vi "VI Tree.vi"   [LabVIEW 2009, in "Keithley 3700 Series.lvlib"]
doc: "This is the instrument driver for the <INSTRUMENT NAME>. The VI Tree displays all the user-callable VIs of the instrument driver in an organized table."
uses:
  <instrlib>/Keithley 3706/Keithley 3700 Series.lvlib
panel:
  # "(c) 2007 <Enter Company Name Here>.  ALL RIGHTS RESERVED."
  # "SEE DIAGRAM\nFOR VI TREE."
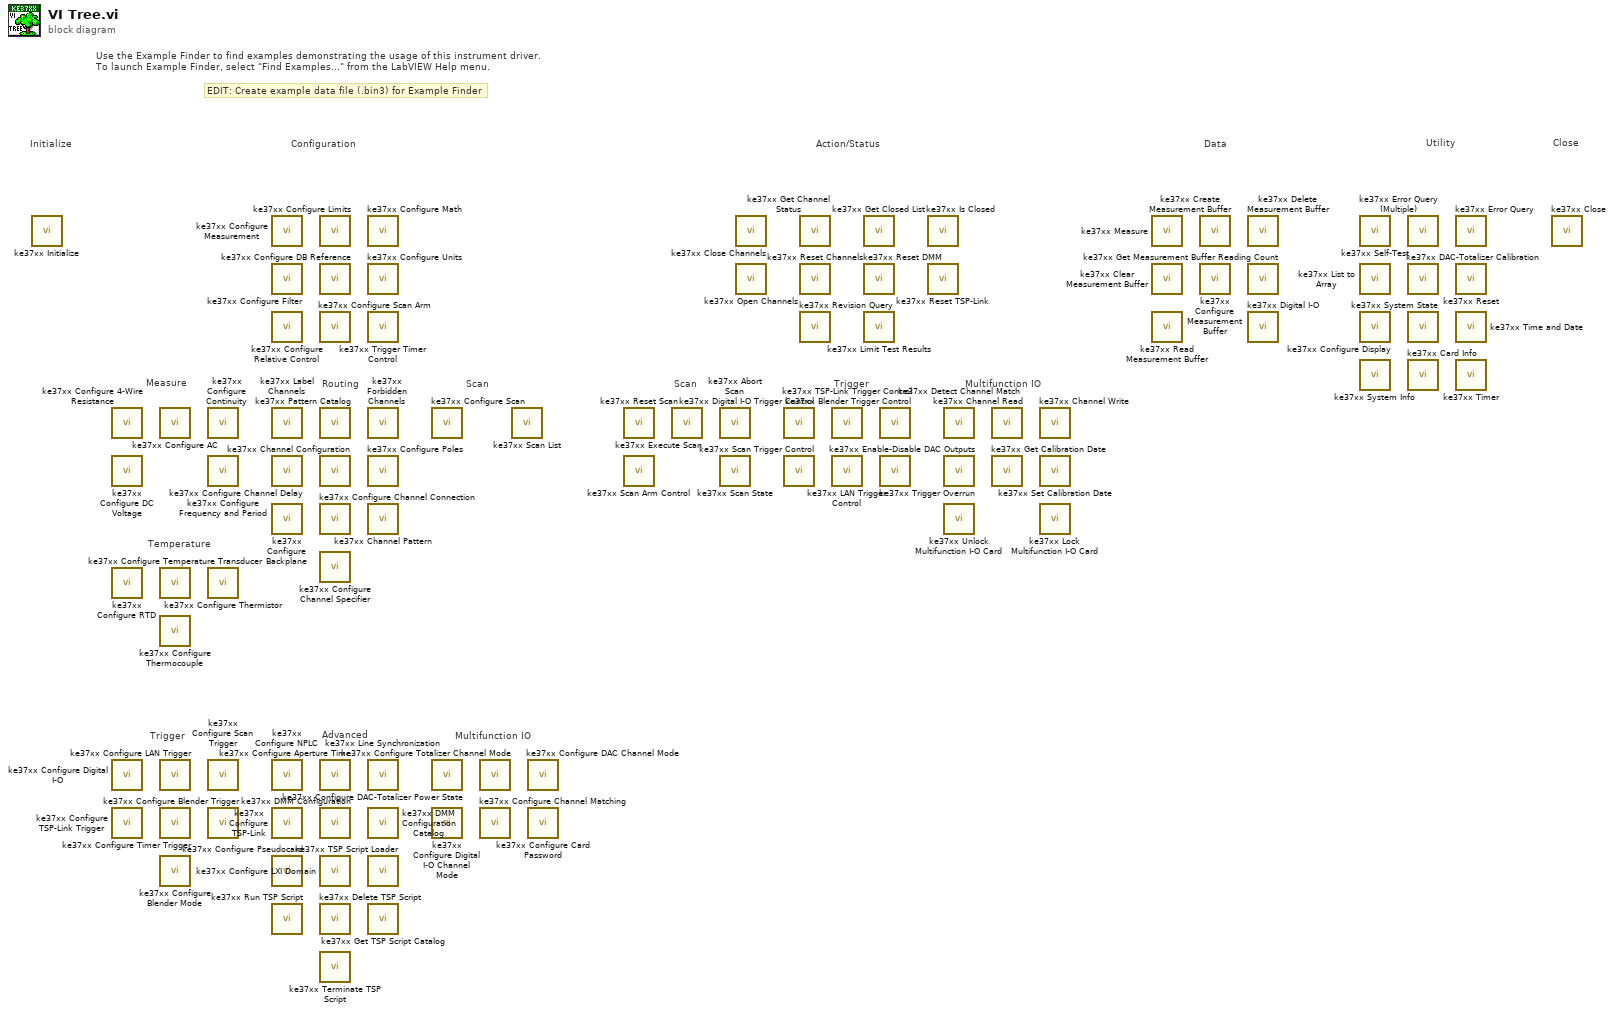
[diagram p0: block diagram]
diagram:
  # "Multifunction IO"
  # "Trigger"
  # "Scan"
  # "Multifunction IO"
  # "Advanced"
  # "Trigger"
  # "Scan"
  # "Routing"
  # "Temperature"
  # "Measure"
  # "EDIT: Create example data file (.bin3) for Example Finder"
  # "Use the Example Finder to find examples demonstrating the usage of this instrument driver.\nTo launch Example Finder, select \"Find Examples...\" from the LabVIEW Help menu."
  # "Configuration"
  # "Utility"
  # "Data"
  # "Action/Status"
  # "Close"
  # "Initialize"
  n1 = call <instrlib>:"ke37xx Initialize.vi"() -> ()  [unwired: 14 in, 2 out]
  n2 = call <instrlib>:"ke37xx Configure 4-Wire Resistance.vi"() -> ()  [unwired: 14 in, 2 out]
  n3 = call <instrlib>:"ke37xx Configure DC Voltage.vi"() -> ()  [unwired: 14 in, 2 out]
  n4 = call <instrlib>:"ke37xx Configure RTD.vi"() -> ()  [unwired: 14 in, 2 out]
  n5 = call <instrlib>:"ke37xx Configure Digital I-O.vi"() -> ()  [unwired: 14 in, 2 out]
  n6 = call <instrlib>:"ke37xx Configure TSP-Link Trigger.vi"() -> ()  [unwired: 14 in, 2 out]
  n7 = call <instrlib>:"ke37xx Configure AC.vi"() -> ()  [unwired: 14 in, 2 out]
  n8 = call <instrlib>:"ke37xx Configure Temperature Transducer.vi"() -> ()  [unwired: 14 in, 2 out]
  n9 = call <instrlib>:"ke37xx Configure Thermocouple.vi"() -> ()  [unwired: 14 in, 2 out]
  n10 = call <instrlib>:"ke37xx Configure LAN Trigger.vi"() -> ()  [unwired: 14 in, 2 out]
  n11 = call <instrlib>:"ke37xx Configure Timer Trigger.vi"() -> ()  [unwired: 14 in, 2 out]
  n12 = call <instrlib>:"ke37xx Configure Blender Mode.vi"() -> ()  [unwired: 14 in, 2 out]
  n13 = call <instrlib>:"ke37xx Configure Continuity.vi"() -> ()  [unwired: 14 in, 2 out]
  n14 = call <instrlib>:"ke37xx Configure Frequency and Period.vi"() -> ()  [unwired: 14 in, 2 out]
  n15 = call <instrlib>:"ke37xx Configure Thermistor.vi"() -> ()  [unwired: 14 in, 2 out]
  n16 = call <instrlib>:"ke37xx Configure Scan Trigger.vi"() -> ()  [unwired: 14 in, 2 out]
  n17 = call <instrlib>:"ke37xx Configure Blender Trigger.vi"() -> ()  [unwired: 14 in, 2 out]
  n18 = call <instrlib>:"ke37xx Configure Measurement.vi"() -> ()  [unwired: 14 in, 2 out]
  n19 = call <instrlib>:"ke37xx Configure Filter.vi"() -> ()  [unwired: 14 in, 2 out]
  n20 = call <instrlib>:"ke37xx Configure Relative Control.vi"() -> ()  [unwired: 14 in, 2 out]
  n21 = call <instrlib>:"ke37xx Label Channels.vi"() -> ()  [unwired: 14 in, 2 out]
  n22 = call <instrlib>:"ke37xx Configure Channel Delay.vi"() -> ()  [unwired: 14 in, 2 out]
  n23 = call <instrlib>:"ke37xx Configure Backplane.vi"() -> ()  [unwired: 14 in, 2 out]
  n24 = call <instrlib>:"ke37xx Configure NPLC.vi"() -> ()  [unwired: 14 in, 2 out]
  n25 = call <instrlib>:"ke37xx Configure TSP-Link.vi"() -> ()  [unwired: 14 in, 2 out]
  n26 = call <instrlib>:"ke37xx Configure Pseudocard.vi"() -> ()  [unwired: 14 in, 2 out]
  n27 = call <instrlib>:"ke37xx Run TSP Script.vi"() -> ()  [unwired: 10 in, 2 out]
  n28 = call <instrlib>:"ke37xx Configure Limits.vi"() -> ()  [unwired: 14 in, 2 out]
  n29 = call <instrlib>:"ke37xx Configure DB Reference.vi"() -> ()  [unwired: 14 in, 2 out]
  n30 = call <instrlib>:"ke37xx Configure Scan Arm.vi"() -> ()  [unwired: 14 in, 2 out]
  n31 = call <instrlib>:"ke37xx Pattern Catalog.vi"() -> ()  [unwired: 13 in, 3 out]
  n32 = call <instrlib>:"ke37xx Channel Configuration.vi"() -> ()  [unwired: 13 in, 3 out]
  n33 = call <instrlib>:"ke37xx Configure Channel Connection.vi"() -> ()  [unwired: 14 in, 2 out]
  n34 = call <instrlib>:"ke37xx Configure Channel Specifier.vi"() -> ()  [unwired: 13 in, 3 out]
  n35 = call <instrlib>:"ke37xx Configure Aperture Time.vi"() -> ()  [unwired: 14 in, 2 out]
  n36 = call <instrlib>:"ke37xx DMM Configuration.vi"() -> ()  [unwired: 13 in, 3 out]
  n37 = call <instrlib>:"ke37xx Configure LXI Domain.vi"() -> ()  [unwired: 14 in, 2 out]
  n38 = call <instrlib>:"ke37xx Delete TSP Script.vi"() -> ()  [unwired: 10 in, 2 out]
  n39 = call <instrlib>:"ke37xx Terminate TSP Script.vi"() -> ()  [unwired: 10 in, 2 out]
  n40 = call <instrlib>:"ke37xx Configure Math.vi"() -> ()  [unwired: 14 in, 2 out]
  n41 = call <instrlib>:"ke37xx Configure Units.vi"() -> ()  [unwired: 14 in, 2 out]
  n42 = call <instrlib>:"ke37xx Trigger Timer Control.vi"() -> ()  [unwired: 13 in, 3 out]
  n43 = call <instrlib>:"ke37xx Forbidden Channels.vi"() -> ()  [unwired: 13 in, 3 out]
  n44 = call <instrlib>:"ke37xx Configure Poles.vi"() -> ()  [unwired: 14 in, 2 out]
  n45 = call <instrlib>:"ke37xx Channel Pattern.vi"() -> ()  [unwired: 13 in, 3 out]
  n46 = call <instrlib>:"ke37xx Line Synchronization.vi"() -> ()  [unwired: 14 in, 2 out]
  n47 = call <instrlib>:"ke37xx DMM Configuration Catalog.vi"() -> ()  [unwired: 13 in, 3 out]
  n48 = call <instrlib>:"ke37xx TSP Script Loader.vi"() -> ()  [unwired: 14 in, 2 out]
  n49 = call <instrlib>:"ke37xx Get TSP Script Catalog.vi"() -> ()  [unwired: 9 in, 3 out]
  n50 = call <instrlib>:"ke37xx Configure Scan.vi"() -> ()  [unwired: 14 in, 2 out]
  n51 = call <instrlib>:"ke37xx Configure DAC-Totalizer Power State.vi"() -> ()  [unwired: 10 in, 2 out]
  n52 = call <instrlib>:"ke37xx Configure Digital I-O Channel Mode.vi"() -> ()  [unwired: 10 in, 2 out]
  n53 = call <instrlib>:"ke37xx Configure Totalizer Channel Mode.vi"() -> ()  [unwired: 10 in, 2 out]
  n54 = call <instrlib>:"ke37xx Configure Channel Matching.vi"() -> ()  [unwired: 14 in, 2 out]
  n55 = call <instrlib>:"ke37xx Scan List.vi"() -> ()  [unwired: 13 in, 3 out]
  n56 = call <instrlib>:"ke37xx Configure DAC Channel Mode.vi"() -> ()  [unwired: 10 in, 2 out]
  n57 = call <instrlib>:"ke37xx Configure Card Password.vi"() -> ()  [unwired: 14 in, 2 out]
  n58 = call <instrlib>:"ke37xx Reset Scan.vi"() -> ()  [unwired: 14 in, 2 out]
  n59 = call <instrlib>:"ke37xx Scan Arm Control.vi"() -> ()  [unwired: 14 in, 2 out]
  n60 = call <instrlib>:"ke37xx Execute Scan.vi"() -> ()  [unwired: 14 in, 2 out]
  n61 = call <instrlib>:"ke37xx Abort Scan.vi"() -> ()  [unwired: 14 in, 2 out]
  n62 = call <instrlib>:"ke37xx Scan State.vi"() -> ()  [unwired: 13 in, 3 out]
  n63 = call <instrlib>:"ke37xx Close Channels.vi"() -> ()  [unwired: 14 in, 2 out]
  n64 = call <instrlib>:"ke37xx Open Channels.vi"() -> ()  [unwired: 14 in, 2 out]
  n65 = call <instrlib>:"ke37xx Digital I-O Trigger Control.vi"() -> ()  [unwired: 13 in, 3 out]
  n66 = call <instrlib>:"ke37xx Scan Trigger Control.vi"() -> ()  [unwired: 14 in, 2 out]
  n67 = call <instrlib>:"ke37xx Get Channel Status.vi"() -> ()  [unwired: 12 in, 4 out]
  n68 = call <instrlib>:"ke37xx Reset Channels.vi"() -> ()  [unwired: 14 in, 2 out]
  n69 = call <instrlib>:"ke37xx Revision Query.vi"() -> ()  [unwired: 8 in, 4 out]
  n70 = call <instrlib>:"ke37xx TSP-Link Trigger Control.vi"() -> ()  [unwired: 13 in, 3 out]
  n71 = call <instrlib>:"ke37xx LAN Trigger Control.vi"() -> ()  [unwired: 13 in, 3 out]
  n72 = call <instrlib>:"ke37xx Get Closed List.vi"() -> ()  [unwired: 13 in, 3 out]
  n73 = call <instrlib>:"ke37xx Reset DMM.vi"() -> ()  [unwired: 14 in, 2 out]
  n74 = call <instrlib>:"ke37xx Limit Test Results.vi"() -> ()  [unwired: 12 in, 4 out]
  n75 = call <instrlib>:"ke37xx Blender Trigger Control.vi"() -> ()  [unwired: 13 in, 3 out]
  n76 = call <instrlib>:"ke37xx Trigger Overrun.vi"() -> ()  [unwired: 13 in, 3 out]
  n77 = call <instrlib>:"ke37xx Is Closed.vi"() -> ()  [unwired: 13 in, 3 out]
  n78 = call <instrlib>:"ke37xx Reset TSP-Link.vi"() -> ()  [unwired: 14 in, 2 out]
  n79 = call <instrlib>:"ke37xx Detect Channel Match.vi"() -> ()  [unwired: 9 in, 3 out]
  n80 = call <instrlib>:"ke37xx Enable-Disable DAC Outputs.vi"() -> ()  [unwired: 10 in, 2 out]
  n81 = call <instrlib>:"ke37xx Unlock Multifunction I-O Card.vi"() -> ()  [unwired: 10 in, 2 out]
  n82 = call <instrlib>:"ke37xx Channel Read.vi"() -> ()  [unwired: 13 in, 3 out]
  n83 = call <instrlib>:"ke37xx Get Calibration Date.vi"() -> ()  [unwired: 9 in, 3 out]
  n84 = call <instrlib>:"ke37xx Channel Write.vi"() -> ()  [unwired: 14 in, 2 out]
  n85 = call <instrlib>:"ke37xx Set Calibration Date.vi"() -> ()  [unwired: 10 in, 2 out]
  n86 = call <instrlib>:"ke37xx Lock Multifunction I-O Card.vi"() -> ()  [unwired: 10 in, 2 out]
  n87 = call <instrlib>:"ke37xx Measure.vi"() -> ()  [unwired: 11 in, 5 out]
  n88 = call <instrlib>:"ke37xx Clear Measurement Buffer.vi"() -> ()  [unwired: 14 in, 2 out]
  n89 = call <instrlib>:"ke37xx Read Measurement Buffer.vi"() -> ()  [unwired: 9 in, 7 out]
  n90 = call <instrlib>:"ke37xx Create Measurement Buffer.vi"() -> ()  [unwired: 14 in, 2 out]
  n91 = call <instrlib>:"ke37xx Configure Measurement Buffer.vi"() -> ()  [unwired: 14 in, 2 out]
  n92 = call <instrlib>:"ke37xx Delete Measurement Buffer.vi"() -> ()  [unwired: 14 in, 2 out]
  n93 = call <instrlib>:"ke37xx Get Measurement Buffer Reading Count.vi"() -> ()  [unwired: 13 in, 3 out]
  n94 = call <instrlib>:"ke37xx Digital I-O.vi"() -> ()  [unwired: 12 in, 4 out]
  n95 = call <instrlib>:"ke37xx Self-Test.vi"() -> ()  [unwired: 12 in, 4 out]
  n96 = call <instrlib>:"ke37xx List to Array.vi"() -> ()  [unwired: 6 in, 2 out]
  n97 = call <instrlib>:"ke37xx Configure Display.vi"() -> ()  [unwired: 14 in, 2 out]
  n98 = call <instrlib>:"ke37xx System Info.vi"() -> ()  [unwired: 11 in, 5 out]
  n99 = call <instrlib>:"ke37xx Error Query (Multiple).vi"() -> ()  [unwired: 12 in, 4 out]
  n100 = call <instrlib>:"ke37xx DAC-Totalizer Calibration.vi"() -> ()  [unwired: 1 in]
  n101 = call <instrlib>:"ke37xx System State.vi"() -> ()  [unwired: 14 in, 2 out]
  n102 = call <instrlib>:"ke37xx Card Info.vi"() -> ()  [unwired: 12 in, 4 out]
  n103 = call <instrlib>:"ke37xx Error Query.vi"() -> ()  [unwired: 12 in, 4 out]
  n104 = call <instrlib>:"ke37xx Reset.vi"() -> ()  [unwired: 14 in, 2 out]
  n105 = call <instrlib>:"ke37xx Time and Date.vi"() -> ()  [unwired: 14 in, 2 out]
  n106 = call <instrlib>:"ke37xx Timer.vi"() -> ()  [unwired: 14 in, 2 out]
  n107 = call <instrlib>:"ke37xx Close.vi"() -> ()  [unwired: 15 in, 1 out]
